vi "Pre-Dig.vi"(8 "Error In":errorcluster, 10 "Selection List[] In":refnum<vi>[](array[refnum]), 11 "VI In":refnum<vi>) -> (0 "Error Out":errorcluster, 2 "Selection List[] Out":refnum<vi>[](array[refnum]), 3 "VI Out":refnum<vi>)   [LabVIEW 2018, in "Tests.lvlib" / "Toolkit.lvlib" / "Integration.lvlib"]
uses:
  Integration.lvlib
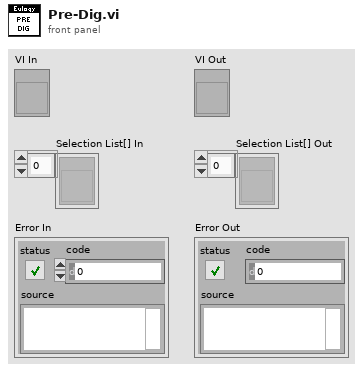
[diagram p1: front panel]
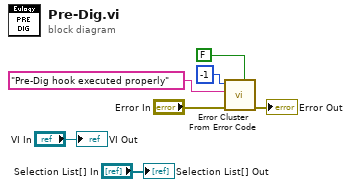
[diagram p0: block diagram]
diagram:
  n1 = call <vilib>:"Error Cluster From Error Code.vi"("is warning? (False)"=FALSE, "error in (no error)"="Error In", "error message (\"\")"="Pre-Dig hook executed properly" ("error message (\"\")"), "error code (0)"=-1) -> ("error out"=→"Error Out":errorcluster)  [unwired: 5 in]
  "Selection List[] Out" <- "Selection List[] In"
  "VI Out" <- "VI In"
